vi "Find and Highlight Event Frames.vi"(8 "error in":errorcluster, 10 "References":refnum<vi>[](array[refnum]), 11 "Event Name":string) -> (0 "error out":errorcluster)   [LabVIEW 2019, in "Panther Dashboard.lvlib"]
uses:
  Panther Dashboard.lvlib
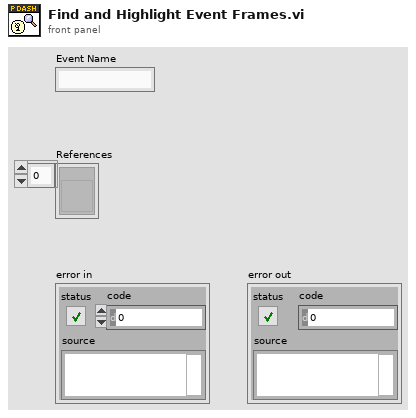
[diagram p1: front panel]
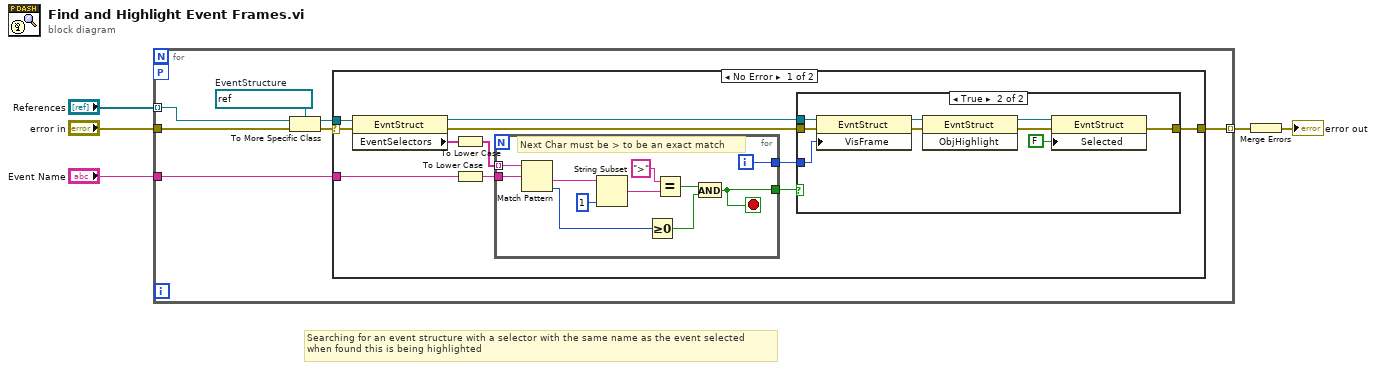
[diagram p0: block diagram]
diagram:
  # "Searching for an event structure with a selector with the same name as the event selected\nwhen found this is being highlighted"
  n1 = for {
    tunnel: "References" -> [w9] mode=indexing
    tunnel: "Event Name" -> [w6]
    tunnel: "error in" -> [w11]
    tunnel: [w10] -> w1 mode=indexing
    workers-P: _ -> [_]
    w8 = refnum<vi> refnum  # EventStructure
    n2 = To More Specific Class(target class=w8, reference=w9, error in=w11) -> (specific class reference=w7:refnum<vi>, error out=w12:errorcluster)
    n3 = case shown="No Error" w12 {
      selector: w12 -> [w23 _]
      tunnel: w7 -> [w18 _]
      tunnel: w6 -> [w19 _]
      tunnel: [w21 _] -> w10
      frame No Error {
        n4 = property class="EvntStruct"(reference=w18, error in=w23) -> (reference out=w15:refnum<vi>, error out=w22:errorcluster, "EventSelectors"=w20:string[])
        n5 = To Lower Case(string=w20) -> (all lower case string=w14:string[])
        n6 = To Lower Case(string=w19) -> (all lower case string=w13:string)
        n7 = for {
          tunnel: w14 -> [w44] mode=indexing
          tunnel: w13 -> [w43]
          tunnel: [w42] -> w17
          tunnel: [w35] -> w16
          i -> [w42]
          stop <- w35 stop-if-true
          # "Next Char must be > to be an exact match"
          n8 = Match Pattern(string=w44, regular expression=w43) -> (after substring=w39:string, offset past match=w40:i32)  [unwired: 1 in, 2 out]
          n9 = String Subset(string=w39, length (rest)=1 ("length (rest)")) -> (substring=w38:string)  [unwired: 1 in]
          n10 = Greater Or Equal To 0?(x=w40) -> (x >= 0?=w41:bool)
          n11 = Equal?(x=">" ("y"), y=w38) -> (x = y?=w36:bool)
          n12 = And(x=w36, y=w41) -> (x .and. y?=w35:bool)
        }
        n13 = case shown="True" w16 {
          tunnel: w15 -> [_ w29]
          tunnel: w17 -> [_ w28]
          tunnel: w22 -> [w24 w32]
          tunnel: [w24 w30] -> w21
          frame False {
          }
          frame True {
            n14 = property class="EvntStruct"(reference=w29, error in=w32, "VisFrame"=w28) -> (reference out=w27:refnum<vi>, error out=w33:errorcluster)
            n15 = invoke class="EvntStruct" method="ObjHighlight"(reference=w27, error in=w33) -> (reference out=w26:refnum<vi>, error out=w31:errorcluster)  [unwired: 1 in, 1 out]
            n16 = property class="EvntStruct"(reference=w26, error in=w31, "Selected"=FALSE) -> (error out=w30:errorcluster)  [unwired: 1 out]
          }
        }
      }
      frame Error {
      }
    }
  }
  n17 = Merge Errors(w1) -> (→"error out":errorcluster)
